vi "FILE Close.vi"(0 "Error In (no error)":errorcluster, 4 "Refnum":refnum<file>) -> (3 "Error Out":errorcluster)   [LabVIEW 2011]
doc: "This VI closes the file for the refnum specified. A close will be attempted regardless of the input error condition."
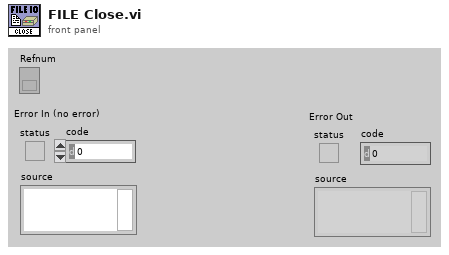
[diagram p1: front panel]
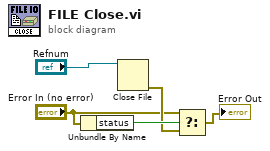
[diagram p0: block diagram]
diagram:
  n1 = Unbundle By Name("Error In (no error)") -> ("status"=w4:bool)
  n2 = Close File(refnum="Refnum") -> (error out=w3:errorcluster)  [unwired: 1 in, 1 out]
  n3 = Select(t="Error In (no error)", s=w4, f=w3) -> (s? t:f=→"Error Out":errorcluster)
